vi "close_driver_session.vi"(7 "Pause after Close (0)":i32, 8 "error in":errorcluster, 11 "VISA resource name":refnum<visa-resource-name>) -> (0 "error out":errorcluster)   [LabVIEW 2014, in "rszvl_rsidr_core.lvlib"]
uses:
  rszvl_rsidr_core.lvlib
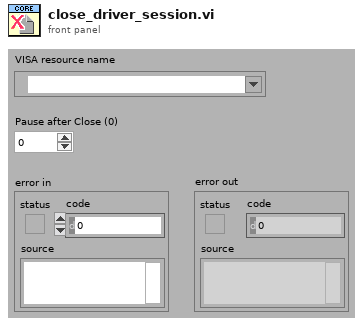
[diagram p1: front panel]
types:
  T1 = enum16{"Initialize", "GetData", "SetData", "Clear"}
  T2 = enum16{"Initialize", "Get Cmd Value", "Reset Rep Cap", "Add Rep Cap", "Remove Rep Cap", "Get Rep Cap ID range", "Get Count", "Clear", "Find Name from NameID", "Get First NameID"}
  T3 = enum16{"Initialize", "Get Cached Value", "Set Cached Value", "Clear"}
  T4 = typedef "rszvl_rsidr_core.lvlib/type_Session_Data.ctl" = cluster{"Instr type":string, "Instr type for err. msg.":string, "Installed Options":string[], "OPC Timeout":i32, "Query Instrument Status":bool, "Check Range":bool, "Check Options":bool, "Add LF to Write":bool, "Simulate":bool, "Logging":bool, "Logging params":variant, "Interface Type":enum16{"Unknown", "GPIB", "VXI", "GPIB_VXI", "ASRL", "PXI", "TCPIP", "USB", "SOCKET"}, "Fast Sweep":i32, "AdditionalFlags":i32, "WaitBeforeWrite":i32, "WaitBeforeRead":i32, "BinDataChunkSize":i64}
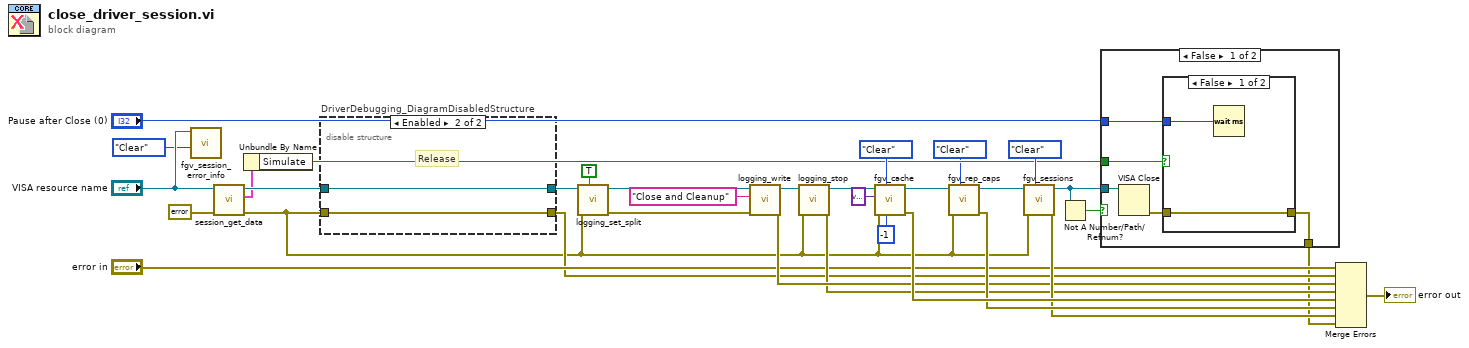
[diagram p0: block diagram]
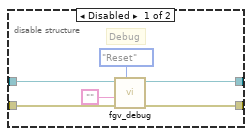
[diagram p2: hidden frame]
diagram:
  n1 = call "fgv_session_error_info.vi"("Operation"=T1."Clear", "Session in"="VISA resource name") -> ()  [unwired: 5 in, 1 out]
  n2 = call "session_get_data.vi"("error in"=errorcluster {"status"=FALSE, "code"=0, "source"=""}, "VISA resource name"="VISA resource name") -> ("error out"=w10:errorcluster, "Session User Data out"=w9:T4, "VISA resource name out"=w12:refnum<visa-resource-name>)  [unwired: 7 in]
  n3 = Unbundle By Name(w9) -> ("Simulate"=w8:bool)
  n4 = disable-structure "DriverDebugging_DiagramDisabledStructure" shown="Enabled" {
    disable-tunnel: w10 -> [w38 w40]
    disable-tunnel: [w36 w40] -> w13
    disable-tunnel: w12 -> [w37 w41]
    disable-tunnel: [w35 w41] -> w15
    frame Disabled {
      # "Debug"
      n5 = call "fgv_debug.vi"("Operation"=enum16{"Reset", "ReadCommand", "SetCommand"}."Reset", "error in"=w38, "Command in"="" ("Empty String Constant"), "VISA resource name"=w37) -> ("error out"=w36:errorcluster, "VISA resource name out"=w35:refnum<visa-resource-name>)  [unwired: 6 in]
    }
    frame Enabled {
      # "Release"
    }
  }
  n6 = call "logging_set_split.vi"("Evaluate section error (F)"=TRUE, "error in"=w10, "VISA resource name"=w15) -> ("error out"=w16:errorcluster, "VISA resource name out"=w3:refnum<visa-resource-name>)  [unwired: 7 in]
  n7 = call "logging_write.vi"("error in"=w16, "String to write"="Close and Cleanup", "VISA resource name"=w3) -> ("error out"=w22:errorcluster, "VISA resource name out"=w18:refnum<visa-resource-name>)  [unwired: 7 in]
  n8 = call "logging_stop.vi"("error in"=w10, "VISA resource name"=w18) -> ("error out"=w21:errorcluster, "VISA resource name out"=w17:refnum<visa-resource-name>)  [unwired: 8 in]
  n9 = call "fgv_cache.vi"("Index in"=-1, "Operation"=T3."Clear" ("Operation (1: Get Cached Value)"), "error in"=w10, "Value in"=variant, "VISA resource name"=w17) -> ("error out"=w30:errorcluster, "VISA resource name out"=w33:refnum<visa-resource-name>)  [unwired: 4 in, 1 out]
  n10 = call "fgv_rep_caps.vi"("Operation"=T2."Clear", "error in"=w10, "VISA resource name"=w33) -> ("error out"=w29:errorcluster, "VISA resource name out"=w20:refnum<visa-resource-name>)  [unwired: 5 in, 2 out]
  n11 = call "fgv_sessions.vi"("Operation"=T1."Clear", "error in"=w10, "VISA resource name"=w20) -> ("error out"=w28:errorcluster, "VISA resource name out"=w19:refnum<visa-resource-name>)  [unwired: 6 in, 1 out]
  n12 = Not A Number/Path/Refnum?(number/path/refnum=w19) -> (NaN/Path/Refnum?=w24:bool)
  n13 = case shown="False" w24 {
    tunnel: w19 -> [w46 _]
    tunnel: w8 -> [w45 _]
    tunnel: [w43 _] -> w7
    tunnel: "Pause after Close (0)" -> [w42 _]
    frame False {
      n14 = VISA Close(VISA resource name=w46) -> (error out=w44:errorcluster)  [unwired: 1 in]
      n15 = case shown="False" w45 {
        tunnel: w44 -> [w48 w49]
        tunnel: [w48 w49] -> w43
        tunnel: w42 -> [w47 _]
        frame False {
          n16 = Wait (ms)(milliseconds to wait=w47) -> ()  [unwired: 1 out]
        }
        frame True {
        }
      }
    }
    frame True {
    }
  }
  n17 = Merge Errors("error in", w13, w22, w21, w30, w29, w28, w7) -> (→"error out":errorcluster)
